vi "20170516-lecture4-2 prof FilterEvent.vi"() -> ()   [LabVIEW 2014]
panel:
  in  "Real Stop Button":bool
  in  "Fake Stop button":bool
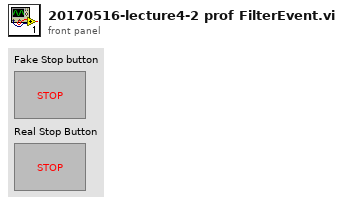
[diagram p1: front panel]
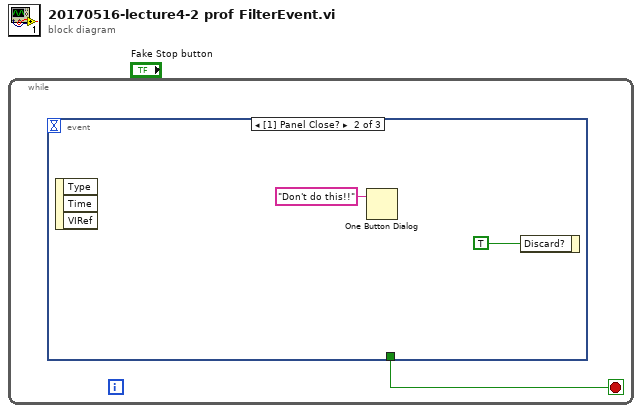
[diagram p0: block diagram]
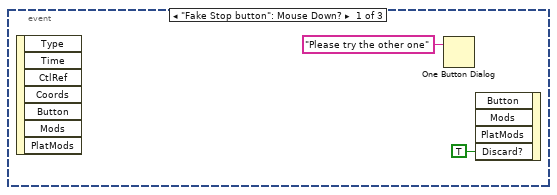
[diagram p2: hidden frame]
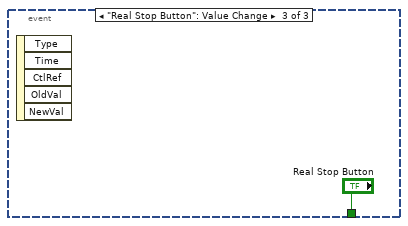
[diagram p3: hidden frame]
diagram:
  n1 = while {
    stop <- w1 stop-if-true
    n2 = event shown="[1] Panel Close?" {
      selector: _ -> [_ _ _]
      dyn-events: _ -> [_ _ _]
      timeout: _ -> [_ _ _]
      tunnel: [_ _ "Real Stop Button"] -> w1
      event "Fake Stop button": Mouse Down? {
        n3 = event-data() -> ()  [unwired: 1 in, 7 out]
        n4 = One Button Dialog(message="Please try the other one") -> ()  [unwired: 1 in, 1 out]
        n5 = event-data("Discard?"=TRUE) -> ()  [unwired: 4 in, 1 out]
      }
      event Panel Close? {
        n6 = event-data() -> ()  [unwired: 1 in, 3 out]
        n7 = One Button Dialog(message="Don't do this!!") -> ()  [unwired: 1 in, 1 out]
        n8 = event-data("Discard?"=TRUE) -> ()  [unwired: 1 in, 1 out]
      }
      event "Real Stop Button": Value Change {
        n9 = event-data() -> ()  [unwired: 1 in, 5 out]
      }
    }
  }
